vi "SetLoCalib.vi"(8 "error in (no error)":errorcluster, 9 "newLoDef":T1, 10 "kParNum":i32, 11 "dvotAFTKinetics in":refnum<class "dvotAFTKinetics.lvclass">) -> (0 "error out":errorcluster, 3 "dvotAFTKinetics out":refnum<class "dvotAFTKinetics.lvclass">)   [LabVIEW 2012, in "dvotAFTKinetics.lvclass"]
uses:
  dvotAFTKinetics.lvclass
  dvotAFTKinetics.lvclass/dvotAFTKinetics.ctl
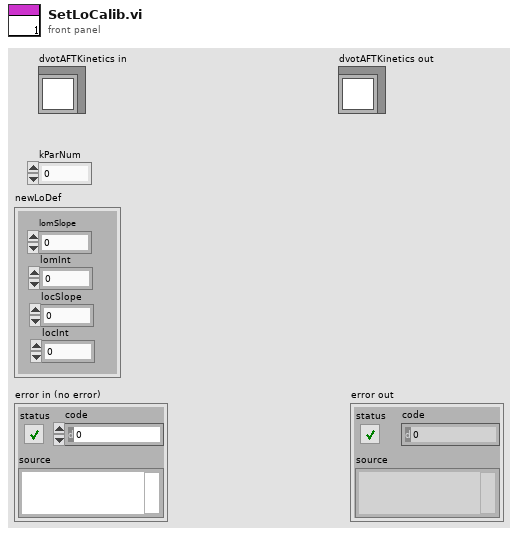
[diagram p1: front panel]
types:
  T1 = cluster{"lomSlope":dbl, "lomInt":dbl, "locSlope":dbl, "locInt":dbl}
  T2 = cluster{"lomSlope":dbl, "lomInt":dbl, "locSlope":dbl, "locInt":dbl}[]
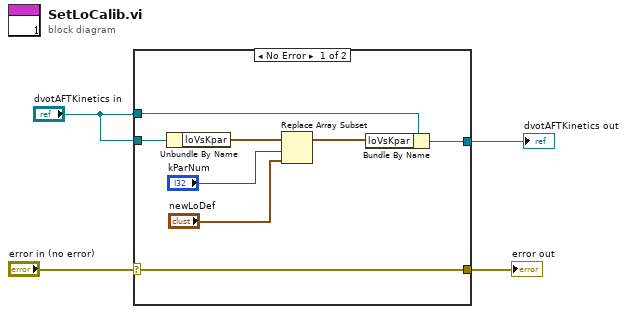
[diagram p0: block diagram]
diagram:
  n1 = case shown="No Error" "error in (no error)" {
    selector: "error in (no error)" -> [w7 w13]
    tunnel: "dvotAFTKinetics in" -> [w12 w14]
    tunnel: [w6 w14] -> w4
    tunnel: [w7 w13] -> w2
    tunnel: "dvotAFTKinetics in" -> [w5 _]
    frame No Error {
      n2 = Unbundle By Name(w12) -> ("loVsKpar"=w11:T2)
      n3 = Replace Array Subset "Replace Array Subset"(array=w11, new element="newLoDef", index="kParNum") -> (w8:T2)
      n4 = Bundle By Name(cluster=w5, "loVsKpar"=w8) -> (w6:refnum<class "dvotAFTKinetics.lvclass">)
    }
    frame Error {
    }
  }
  "dvotAFTKinetics out" <- w4
  "error out" <- w2
